vi "AMI Payload Parse.vi"(11 "Payload":string) -> (1 "Version-Revision":string, 2 "Model Name":string, 3 "Information":string)   [LabVIEW 2015, in "Samwontech TEMP2xxx.lvlib"]
uses:
  Samwontech TEMP2xxx.lvlib
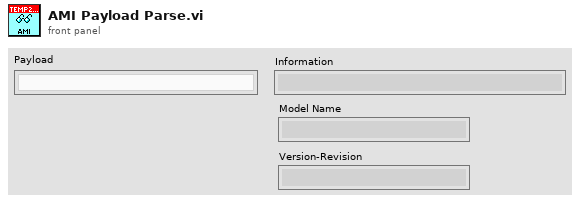
[diagram p1: front panel]
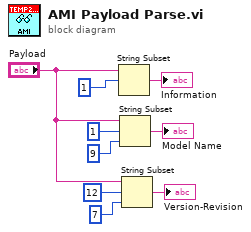
[diagram p0: block diagram]
diagram:
  n1 = String Subset(string="Payload", offset (0)=1) -> (substring=→"Information":string)  [unwired: 1 in]
  n2 = String Subset(string="Payload", offset (0)=1, length (rest)=9 ("length (rest)")) -> (substring=→"Model Name":string)
  n3 = String Subset(string="Payload", offset (0)=12, length (rest)=7 ("length (rest)")) -> (substring=→"Version-Revision":string)
